vi "MegaAwesome_8_29_12c_JW.vi"() -> ()   [LabVIEW 2011]
uses:
  MegaAwesome_States.ctl
  <vilib>/Utility/file.llb/Read From Spreadsheet File (string).vi
  <vilib>/Utility/file.llb/Write To Spreadsheet File (string).vi
panel:
  in  "Index-Sat":dbl=5.0
  in  "Index-Lin":dbl=5.0
  in  "IndexLog-Lin":dbl=5.0
  in  "IndexLog-Sat":dbl=5.0 caption="Num Pts"
  out "Lin Id-Log Used":dbl[](array[numeric])
  out "Lin-Vg Array-Log Used":dbl[](array[numeric])
  out "Total Width":dbl
  out "Image Preview":T1(plugin-control)
  in  "New: Comments":string
  out "Save Array":string[][](array[string])
  out "Folder Index":i32 caption="Length"
  out "Sat Id-Used":dbl[](array[numeric])
  out "Sat Vg Array-Used":dbl[](array[numeric])
  out "Vg Array-Log-Used":dbl[](array[numeric])
  out "Sat Id-Log-Used":dbl[](array[numeric])
  out "Lin Id-Used":dbl[](array[numeric])
  out "Lin-Vg Array-Used":dbl[](array[numeric])
  out "Lin Vd":dbl
  out "Recorded Prop":T2
  out "Current State":T3
  in  "Main Tab Control":T4(tab)
  in  "Image Folder":path
  out "Image File":path=path "D:/UserData/Desktop/Jeremy/WFU/Research/Programs/VI mods/Image Not Found.png"
  in  "Transfer File":path
  out "Transfer Folder":path
  out "Fabrication Prop":T5
  in  "Manual Controls":T6
  in  "File Controls":T7
  out "Date Recorded":string="Date Recorded" caption="Measured"
  out "Data Name:":string
  out "Image Name":string
  out "Index":string
  out "Date Created":string caption="Fabricated"
  in  "Comments:":string
  out "Rec: Length":dbl caption="Length" format="%#_3g"
  out "Rec: Width":dbl caption="Width" format="%#_4g"
  out "Rec: Dielectric (d)":dbl caption="Dielectric (d)" format="%#_3g"
  in  "New: Dielectric":dbl
  in  "New: Length":dbl
  in  "New: Width":dbl
  out "Rec: Temp":dbl caption="Sample Temp" format="%.1f"
  in  "New: Temp":dbl format="%.1f"
  in  "Independant Variable":string(combo)="Length (um):"
  out "Image Out":T1(plugin-control)
  in  "Num Pts":dbl=5.0
  in  "Num Pts Log":dbl=5.0 caption="Num Pts"
  out "Recorded Values Cluster":T8
  out "Calculated Values Cluster":T8 caption="Recorded Values Cluster"
  out "Re-Calculated Values Cluster":T8 caption="Recorded Values Cluster"
  in  "Origin Project File":path=path "\\\\acad1\\physics/Jurchescu-group/JW-PD/Group Library/Origin Project Files/DeviceData_8_10_12a_JW.opj"
  in  "No Image File":path=path "\\\\acad1\\physics/Jurchescu-group/JW-PD/Mega Awesome/Image Not Found.png"
  in  "Room Temp":dbl=294.0
  # "Image Location"
  # "Recorded"
  # "Calculated"
  # "Re-Calculated"
  # "Manual"
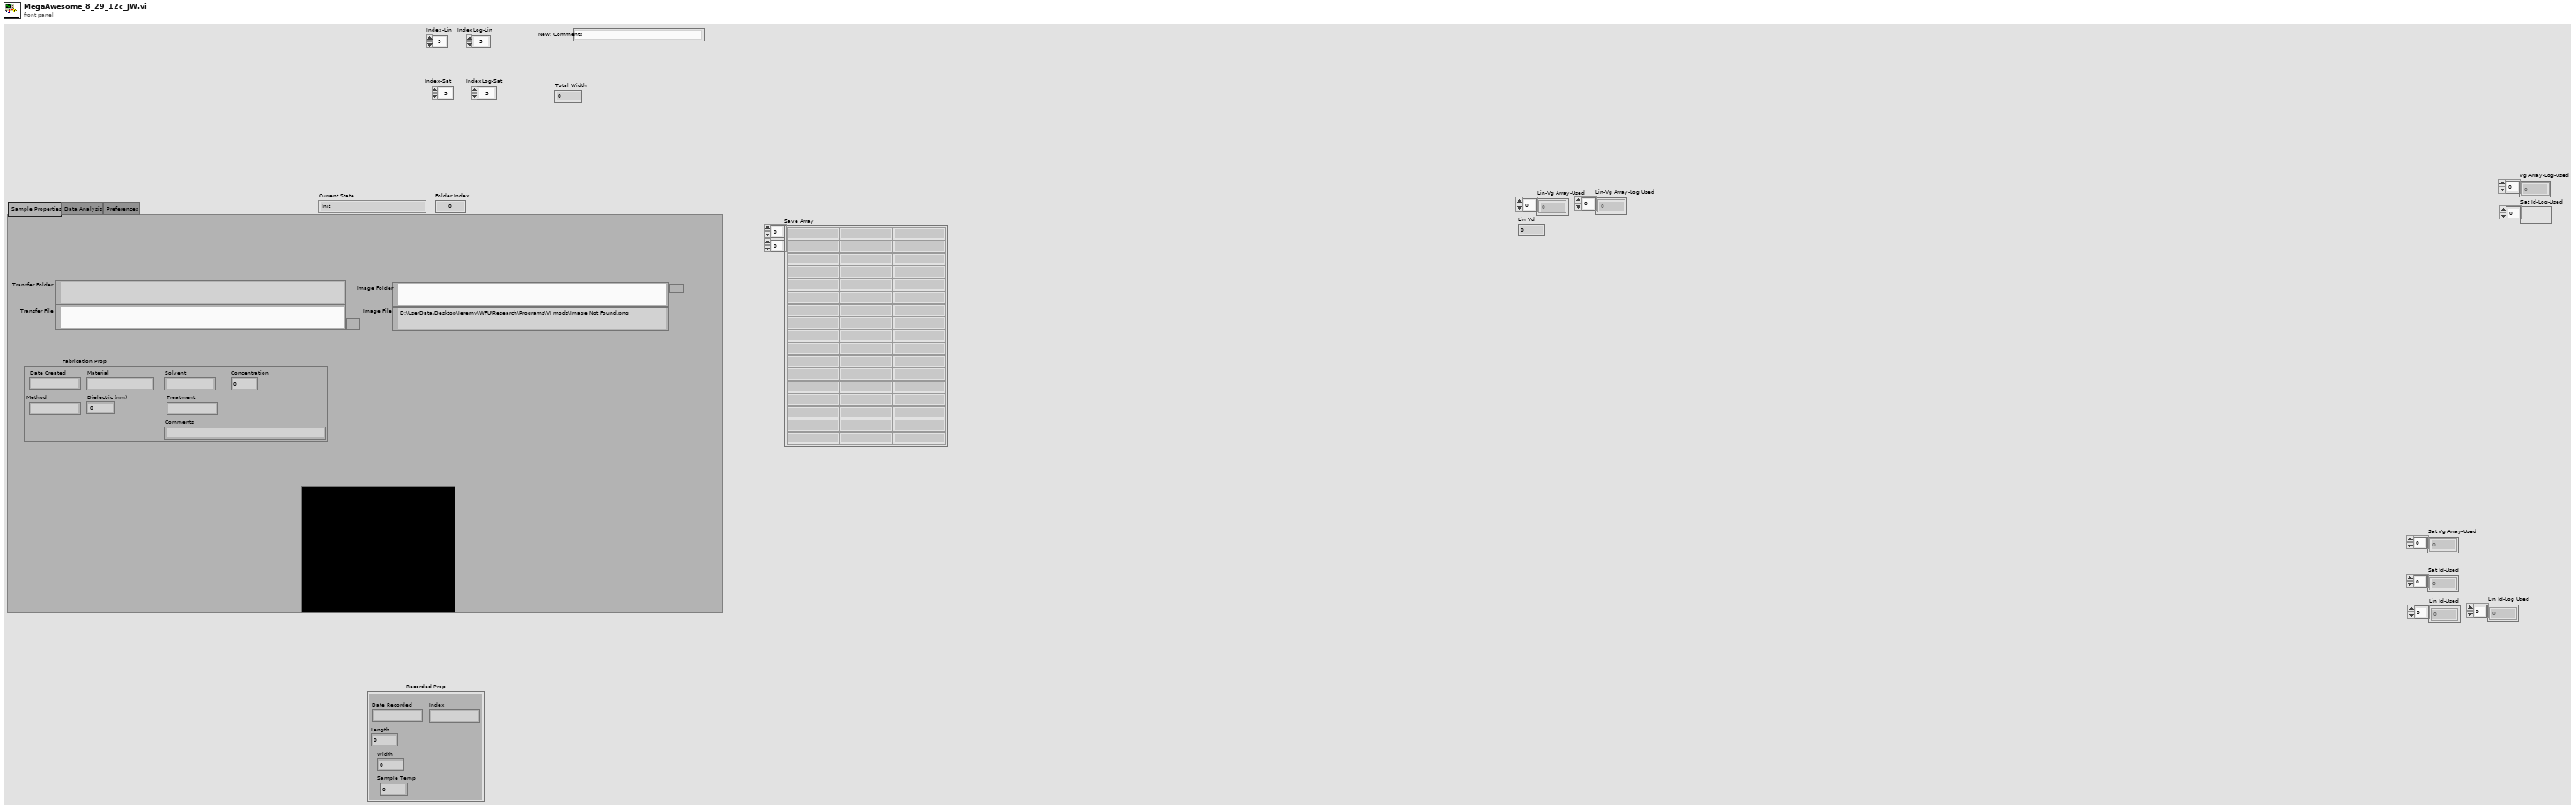
[diagram p1: front panel]
types:
  T1 = typedef "IMAQ Image.ctl" = refnum<image>
  T2 = cluster{"Date Recorded":string, "Index":string, "Length":dbl, "Width":dbl, "Sample Temp":dbl}
  T3 = typedef "MegaAwesome_States.ctl" = enum16{"Init", "File Missing", "No Event", "Read Data", "Calculated Values", "Re-Calculated Values", "Next File", "Previous File", "Discard File", "Save", "Save Lines", "Export", "Exit"}
  T4 = enum32{"Sample Properties", "Data Analysis", "Preferences"}
  T5 = cluster{"Date Created":string, "Material":string, "Solvent":string, "Concentration":dbl, "Method":string, "Dielectric (nm)":dbl, "Treatment":string, "Comments":string}
  T6 = cluster{"Manual-Temp":bool, "Manual-Width":bool, "Manuel-Length":bool, "Manuel-Dielectric":bool, "Manual Comments":bool}
  T7 = cluster{"Previous File":bool, "Discard ":bool, "Save Lines":bool, "Close":bool, "Next File ":bool, "Save":bool, "Save Next":bool, "Export":bool}
  T8 = cluster{"Mobility-Sat":dbl, "Moblitity-Lin":dbl, "On/Off":dbl, "Off Current":dbl, "Vt-Sat":dbl, "STS":dbl, "Trap Density-VT":dbl, "Trap Density-STS":dbl}
  T9 = cluster{"Sat Vg Used":dbl[], "Sat Sqrt(Id) Used ":dbl[], "Lin Vg Used":dbl[], "Lin Sqrt(Id) Used":dbl[], "Index-Lin":dbl, "Index-Sat":dbl}
  T10 = cluster{"Mobility-Sat":dbl, "Vt-Sat":dbl, "Mobility-Lin":dbl, "Vt-Lin":dbl, "Off I-Sat":dbl, "On/Off I-Sat":dbl}
  T11 = cluster{"Sat Vg Used":dbl[], "Sat Log(Id) Used":dbl[], "Lin Vg Used":dbl[], "Lin Log(Id) Used":dbl[], "STS Index-Sat":dbl, "STS Index-Lin":dbl}
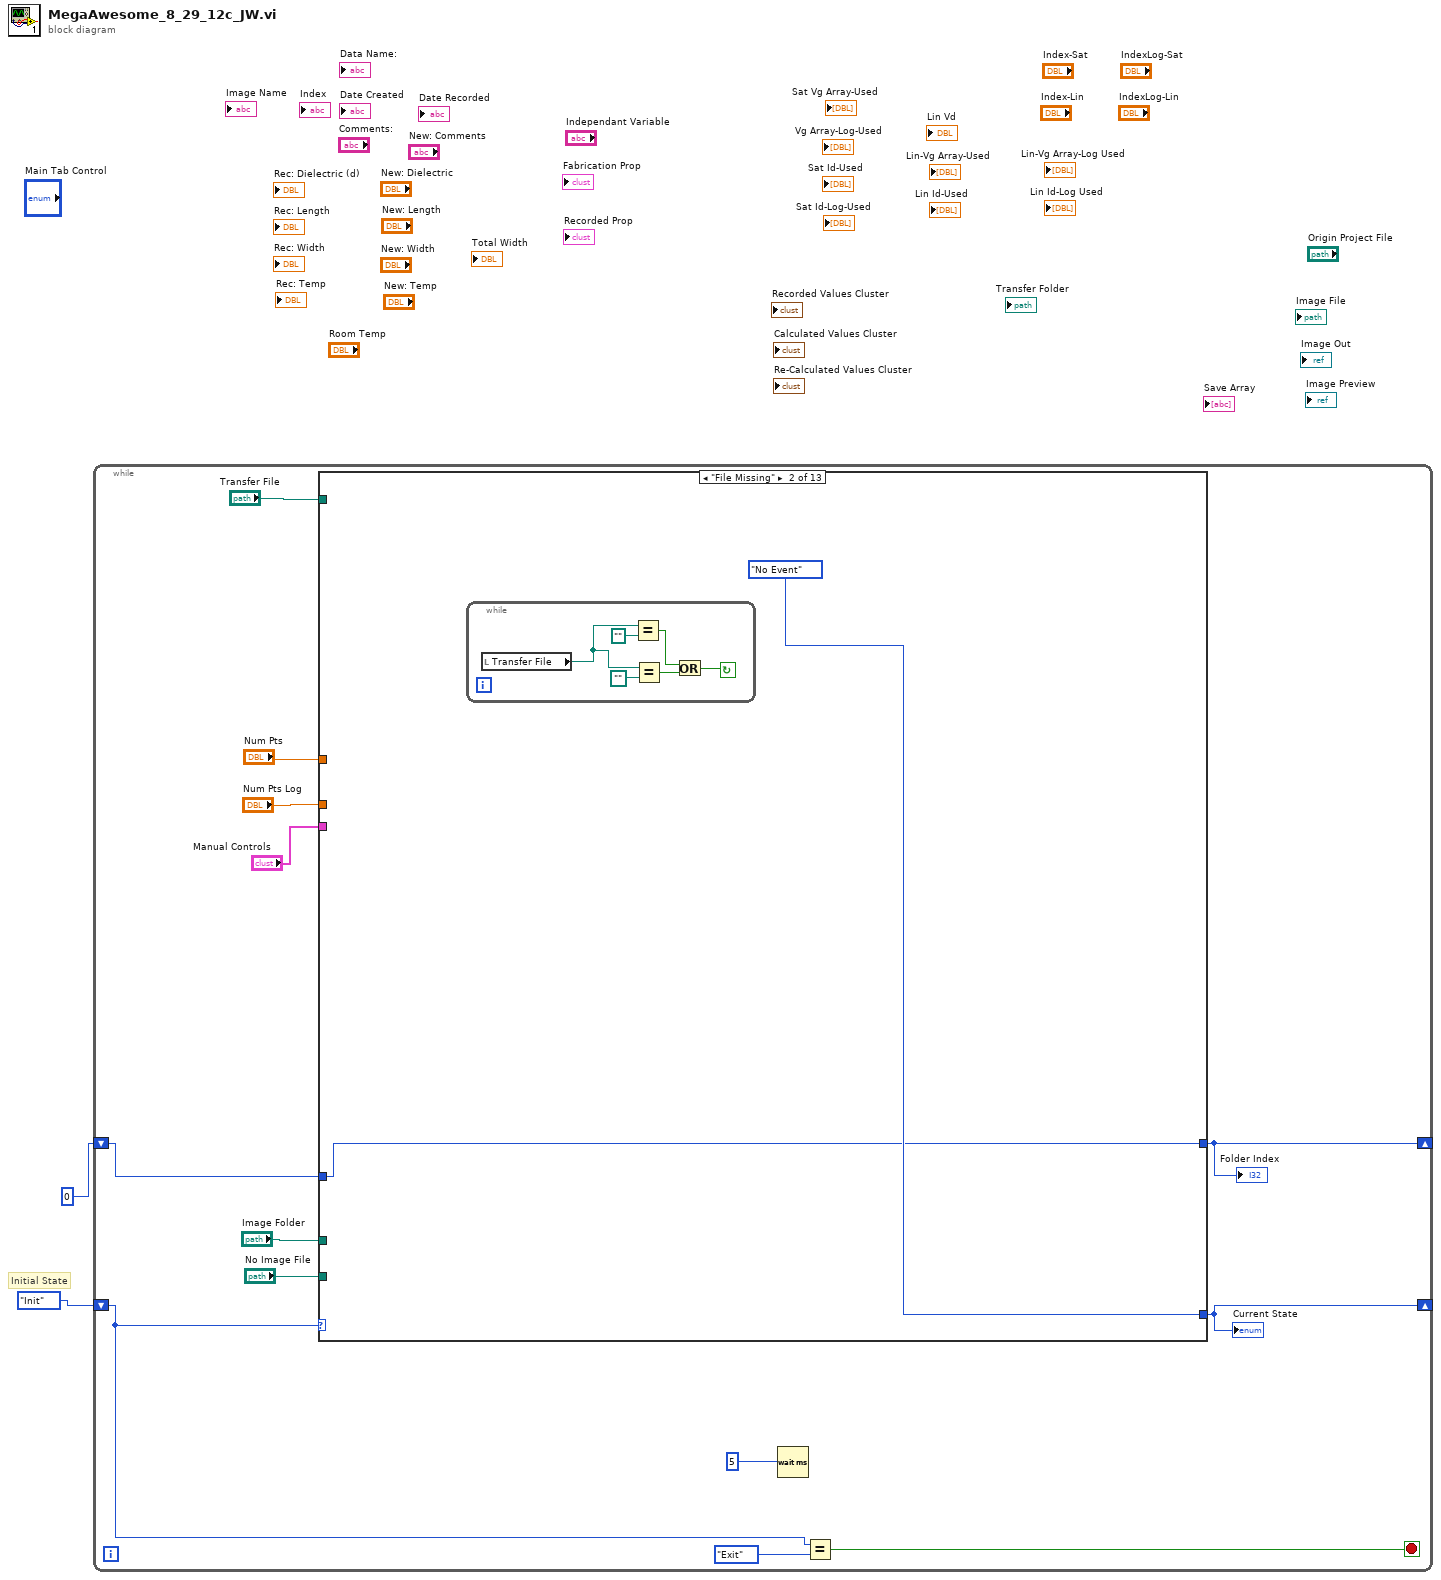
[diagram p0: block diagram]
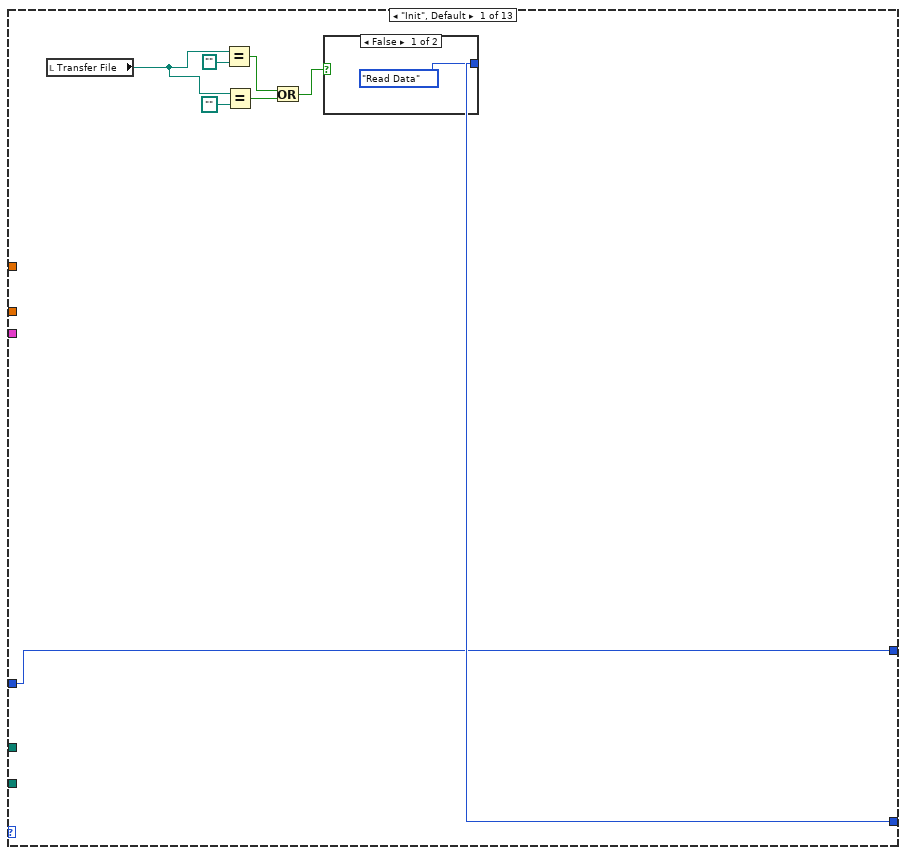
[diagram p2: hidden frame]
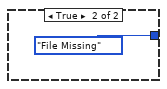
[diagram p3: hidden frame]
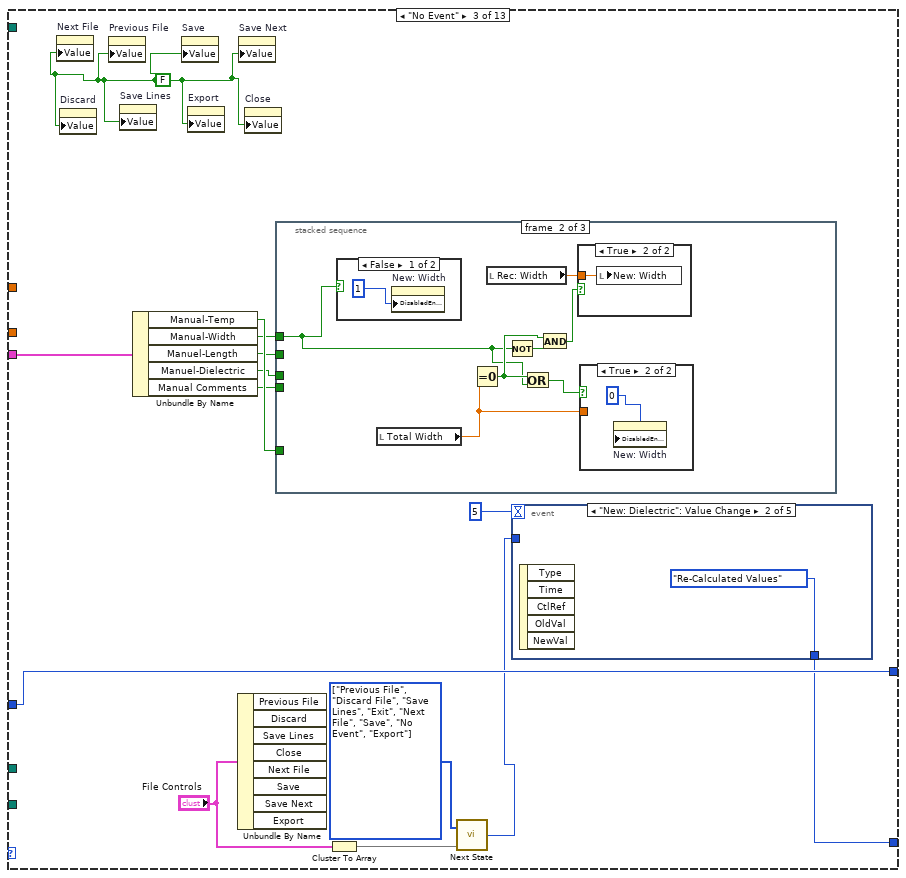
[diagram p4: hidden frame]
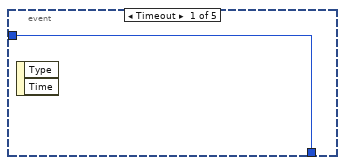
[diagram p5: hidden frame]
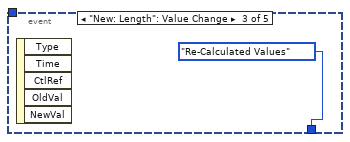
[diagram p6: hidden frame]
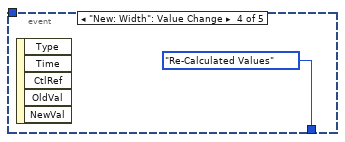
[diagram p7: hidden frame]
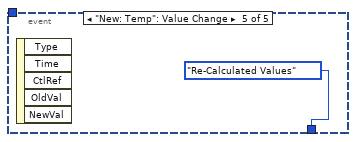
[diagram p8: hidden frame]
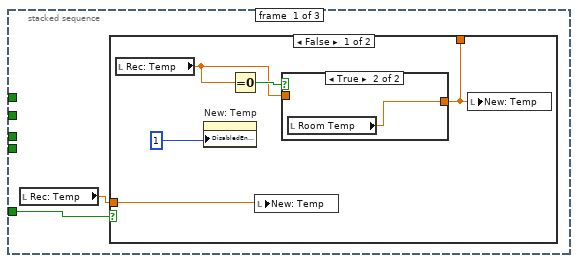
[diagram p9: hidden frame]
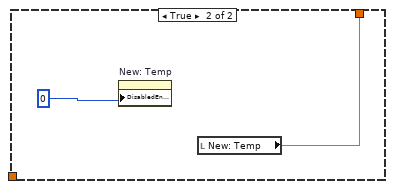
[diagram p11: hidden frame]
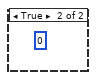
[diagram p12: hidden frame]
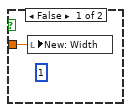
[diagram p14: hidden frame]
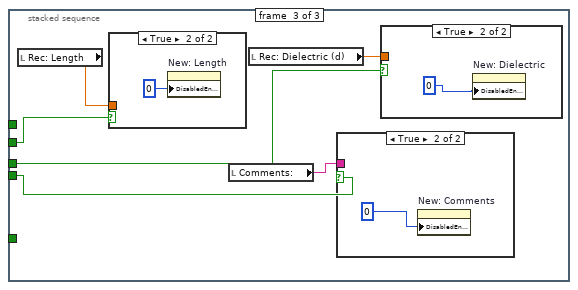
[diagram p15: hidden frame]
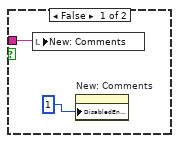
[diagram p16: hidden frame]
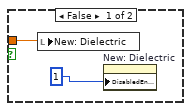
[diagram p17: hidden frame]
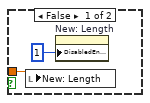
[diagram p18: hidden frame]
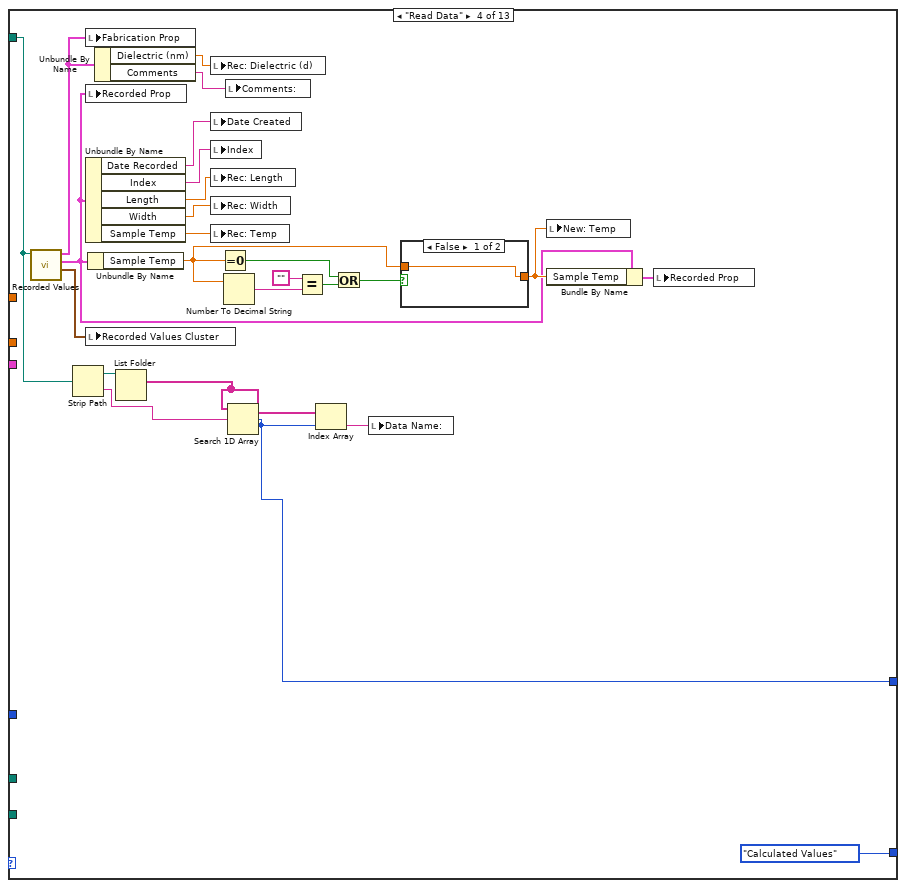
[diagram p19: hidden frame]
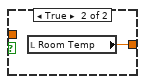
[diagram p20: hidden frame]
diagram:
  # "Initial State"
  n1 = while {
    shift-right: [w12] -> _
    shift-left: MegaAwesome_States."Init" -> [w14]
    shift-right: [w5] -> _
    shift-left: 0 -> [w6]
    stop <- w15 stop-if-true
    n2 = case shown="\"File Missing\"" w14 {
      selector: w14 -> [_ _ _ _ _ _ _ w210 _ _ _ _ _]
      tunnel: [w17 MegaAwesome_States."No Event" w35 MegaAwesome_States."Calculated Values" MegaAwesome_States."Re-Calculated Values" MegaAwesome_States."No Event" MegaAwesome_States."Read Data" w210 MegaAwesome_States."Read Data" MegaAwesome_States."No Event" w235 MegaAwesome_States."No Event" MegaAwesome_States."No Event"] -> w12
      tunnel: "Transfer File" -> [_ _ _ w96 w135 _ w203 _ w217 _ w240 _ _]
      tunnel: "Num Pts" -> [_ _ _ _ w139 _ _ _ _ _ _ _ _]
      tunnel: "Num Pts Log" -> [_ _ _ _ w138 _ _ _ _ _ _ _ _]
      tunnel: "Image Folder" -> [_ _ _ _ w134 _ _ _ _ _ _ _ _]
      tunnel: "No Image File" -> [_ _ _ _ w133 _ _ _ _ _ _ _ _]
      tunnel: [w16 w26 w43 w90 w132 w163 w188 w209 w215 w233 w241 w752 w754] -> w5
      tunnel: w6 -> [w16 w26 w43 _ w132 w163 w189 w209 w216 w233 w241 w752 w754]
      tunnel: "Manual Controls" -> [_ _ w37 _ _ _ _ _ _ _ w239 _ _]
      frame "Init", Default {
        n3 = local read "Transfer File"() -> (w18:path)
        n4 = Equal?(x=w18, y=path "") -> (x = y?=w21:bool)
        n5 = Equal?(x=w18, y=path "") -> (x = y?=w20:bool)
        n6 = Or(x=w21, y=w20) -> (x .or. y?=w23:bool)
        n7 = case shown="False" w23 {
          tunnel: [MegaAwesome_States."Read Data" MegaAwesome_States."File Missing"] -> w17
          frame False {
          }
          frame True {
          }
        }
      }
      frame "File Missing" {
        n8 = while {
          stop <- w28 continue-if-true
          n9 = local read "Transfer File"() -> (w29:path)
          n10 = Equal?(x=w29, y=path "") -> (x = y?=w31:bool)
          n11 = Equal?(x=w29, y=path "") -> (x = y?=w32:bool)
          n12 = Or(x=w31, y=w32) -> (x .or. y?=w28:bool)
        }
      }
      frame "No Event" {
        w46 = T3[] [enum."Previous File", enum."Discard File", enum."Save Lines", enum."Exit", enum."Next File", enum."Save", enum."No Event", enum."Export"] items=["Init", "File Missing", "No Event", "Read Data", "Calculated Values", "Re-Calculated Values", "Next File", "Previous File", "Discard File", "Save", "Save Lines", "Export", "Exit"]
        w47 = FALSE
        n13 = property on="Next File" class="Bool (strict)"("Value"=w47) -> ()  [unwired: 2 in, 2 out]
        n14 = property on="Discard" class="Bool (strict)"("Value"=w47) -> ()  [unwired: 2 in, 2 out]
        n15 = property on="Previous File" class="Bool (strict)"("Value"=w47) -> ()  [unwired: 2 in, 2 out]
        n16 = property on="Save Lines" class="Bool (strict)"("Value"=w47) -> ()  [unwired: 2 in, 2 out]
        n17 = Unbundle By Name(w37) -> ("Manual-Temp"=w42:bool, "Manual-Width"=w41:bool, "Manuel-Length"=w40:bool, "Manuel-Dielectric"=w39:bool, "Manual Comments"=w38:bool)
        n18 = property on="Save" class="Bool (strict)"("Value"=w47) -> ()  [unwired: 2 in, 2 out]
        n19 = property on="Export" class="Bool (strict)"("Value"=w47) -> ()  [unwired: 2 in, 2 out]
        n20 = Unbundle By Name("File Controls") -> ()  [unwired: 8 out]
        n21 = property on="Save Next" class="Bool (strict)"("Value"=w47) -> ()  [unwired: 2 in, 2 out]
        n22 = property on="Close" class="Bool (strict)"("Value"=w47) -> ()  [unwired: 2 in, 2 out]
        n23 = stacked-sequence {
          tunnel: w42 -> [w54 _ _]
          tunnel: w41 -> [_ w64 _]
          tunnel: w40 -> [_ _ w79]
          tunnel: w39 -> [_ _ w76]
          tunnel: w38 -> [_ _ w75]
          frame #0 {
            n24 = local read "Rec: Temp"() -> (w53:dbl)
            n25 = case shown="False" w54 {
              tunnel: w53 -> [w59 _]
              tunnel: [w56 w63] -> _
              frame False {
                n26 = local read "Rec: Temp"() -> (w57:dbl)
                n27 = property on="New: Temp" class="DigNum (strict)"("DisabledEnum"=1) -> ()  [unwired: 2 in, 2 out]
                n28 = Equal To 0?(x=w57) -> (x = 0?=w58:bool)
                n29 = local write "New: Temp"(w59) -> ()
                n30 = case shown="True" w58 {
                  tunnel: [w60 w61] -> w56
                  tunnel: w57 -> [w60 _]
                  frame False {
                  }
                  frame True {
                    n31 = local read "Room Temp"() -> (w61:dbl)
                  }
                }
                n32 = local write "New: Temp"(w56) -> ()
              }
              frame True {
                n33 = property on="New: Temp" class="DigNum (strict)"("DisabledEnum"=0) -> ()  [unwired: 2 in, 2 out]
                n34 = local read "New: Temp"() -> (w63:dbl)
              }
            }
          }
          frame #1 {
            n35 = case shown="False" w64 {
              frame False {
                n36 = property on="New: Width" class="DigNum (strict)"("DisabledEnum"=1) -> ()  [unwired: 2 in, 2 out]
              }
              frame True {
                (unwired) 0
              }
            }
            n37 = local read "Total Width"() -> (w70:dbl)
            n38 = Equal To 0?(x=w70) -> (x = 0?=w67:bool)
            n39 = local read "Rec: Width"() -> (w68:dbl)
            n40 = Not(x=w64) -> (.not. x?=w66:bool)
            n41 = Or(x=w67, y=w64) -> (x .or. y?=w69:bool)
            n42 = And(x=w67, y=w66) -> (x .and. y?=w65:bool)
            n43 = case shown="True" w65 {
              tunnel: w68 -> [_ w72]
              frame False {
              }
              frame True {
                n44 = local write "New: Width"(w72) -> ()
              }
            }
            n45 = case shown="True" w69 {
              tunnel: w70 -> [w73 _]
              frame False {
                (unwired) 1
                n46 = local write "New: Width"(w73) -> ()
              }
              frame True {
                n47 = property on="New: Width" class="DigNum (strict)"("DisabledEnum"=0) -> ()  [unwired: 2 in, 2 out]
              }
            }
          }
          frame #2 {
            n48 = local read "Rec: Length"() -> (w80:dbl)
            n49 = case shown="True" w79 {
              tunnel: w80 -> [w88 _]
              frame False {
                n50 = local write "New: Length"(w88) -> ()
                n51 = property on="New: Length" class="DigNum (strict)"("DisabledEnum"=1) -> ()  [unwired: 2 in, 2 out]
              }
              frame True {
                n52 = property on="New: Length" class="DigNum (strict)"("DisabledEnum"=0) -> ()  [unwired: 2 in, 2 out]
              }
            }
            n53 = local read "Comments:"() -> (w77:string)
            n54 = local read "Rec: Dielectric (d)"() -> (w78:dbl)
            n55 = case shown="True" w75 {
              tunnel: w77 -> [w82 _]
              frame False {
                n56 = local write "New: Comments"(w82) -> ()
                n57 = property on="New: Comments" class="Str"("DisabledEnum"=1) -> ()  [unwired: 2 in, 2 out]
              }
              frame True {
                n58 = property on="New: Comments" class="Str"("DisabledEnum"=0) -> ()  [unwired: 2 in, 2 out]
              }
            }
            n59 = case shown="True" w76 {
              tunnel: w78 -> [w85 _]
              frame False {
                n60 = local write "New: Dielectric"(w85) -> ()
                n61 = property on="New: Dielectric" class="DigNum (strict)"("DisabledEnum"=1) -> ()  [unwired: 2 in, 2 out]
              }
              frame True {
                n62 = property on="New: Dielectric" class="DigNum (strict)"("DisabledEnum"=0) -> ()  [unwired: 2 in, 2 out]
              }
            }
          }
        }
        n63 = Cluster To Array(cluster="File Controls") -> (array=w44:bool[])
        n64 = call "Next State.vi"("Buttons []"=w44, "States []"=w46) -> ("Enum"=w36:T3)
        n65 = event shown="[1] \"New: Dielectric\": Value Change" {
          selector: _ -> [_ _ _ _ _]
          dyn-events: _ -> [_ _ _ _ _]
          timeout: 5 -> [_ _ _ _ _]
          tunnel: w36 -> [w48 _ _ _ _]
          tunnel: [w48 MegaAwesome_States."Re-Calculated Values" MegaAwesome_States."Re-Calculated Values" MegaAwesome_States."Re-Calculated Values" MegaAwesome_States."Re-Calculated Values"] -> w35
          event Timeout {
            n66 = event-data() -> ()  [unwired: 1 in, 2 out]
          }
          event "New: Dielectric": Value Change {
            n67 = event-data() -> ()  [unwired: 1 in, 5 out]
          }
          event "New: Length": Value Change {
            n68 = event-data() -> ()  [unwired: 1 in, 5 out]
          }
          event "New: Width": Value Change {
            n69 = event-data() -> ()  [unwired: 1 in, 5 out]
          }
          event "New: Temp": Value Change {
            n70 = event-data() -> ()  [unwired: 1 in, 5 out]
          }
        }
      }
      frame "Read Data" {
        n71 = call "Recorded Values.vi"("Path"=w96) -> ("Recorded Char"=w114:T8, "Recorded Prop"=w104:T2, "Fabrication Prop"=w98:T5)  [unwired: 8 in]
        n72 = Strip Path(path=w96) -> (stripped path=w97:path, name=w95:string)
        n73 = local write "Fabrication Prop"(w98) -> ()
        n74 = local write "Recorded Prop"(w104) -> ()
        n75 = Unbundle By Name(w104) -> ("Date Recorded"=w103:string, "Index"=w101:string, "Length"=w102:dbl, "Width"=w100:dbl, "Sample Temp"=w99:dbl)
        n76 = local write "Recorded Values Cluster"(w114) -> ()
        n77 = Unbundle By Name(w104) -> ("Sample Temp"=w107:dbl)
        n78 = Unbundle By Name(w98) -> ("Dielectric (nm)"=w92:dbl, "Comments"=w91:string)
        n79 = List Folder(path=w97) -> (filenames=w93:string[])  [unwired: 3 in, 3 out]
        n80 = local write "Rec: Dielectric (d)"(w92) -> ()
        n81 = local write "Date Created"(w103) -> ()
        n82 = local write "Index"(w101) -> ()
        n83 = local write "Rec: Length"(w102) -> ()
        n84 = local write "Rec: Width"(w100) -> ()
        n85 = local write "Rec: Temp"(w99) -> ()
        n86 = Equal To 0?(x=w107) -> (x = 0?=w110:bool)
        n87 = Number To Decimal String(number=w107) -> (decimal integer string=w111:string)  [unwired: 1 in]
        n88 = local write "Comments:"(w91) -> ()
        n89 = Search 1D Array(1D array=w93, element=w95) -> (index of element=w90:i32)  [unwired: 1 in]
        n90 = Equal?(x="", y=w111) -> (x = y?=w109:bool)
        n91 = Index Array(array=w93, index=w90) -> (element=w94:string)
        n92 = Or(x=w110, y=w109) -> (x .or. y?=w108:bool)
        n93 = local write "Data Name:"(w94) -> ()
        n94 = case shown="False" w108 {
          tunnel: [w115 w116] -> w105
          tunnel: w107 -> [w115 _]
          frame False {
          }
          frame True {
            n95 = local read "Room Temp"() -> (w116:dbl)
          }
        }
        n96 = local write "New: Temp"(w105) -> ()
        n97 = Bundle By Name(cluster=w104, "Sample Temp"=w105) -> (w106:T2)
        n98 = local write "Recorded Prop"(w106) -> ()
      }
      frame "Calculated Values" {
        n99 = local read "Fabrication Prop"() -> (w144:T5)
        n100 = local read "Recorded Prop"() -> (w137:T2)
        n101 = disable-structure shown="Disabled" {
          disable-tunnel: w135 -> [w161 _]
          disable-tunnel: w134 -> [w160 _]
          disable-tunnel: w133 -> [w159 _]
          frame Disabled {
            n102 = call "Image from TRF Display.vi"("No Image File"=w159, "Image Folder"=w160, "Transfer File"=w161) -> ("Image Out 2"=w155:T1, "Image Out"=w156:T1, "Image File"=w157:path, "Image Name"=w158:string)  [unwired: 5 in]
            n103 = local write "Image Name"(w158) -> ()
            n104 = local write "Image File"(w157) -> ()
            n105 = local write "Image Out"(w156) -> ()
            n106 = local write "Image Preview"(w155) -> ()
          }
          frame Enabled {
          }
        }
        n107 = local read "Calculated Values Cluster"() -> (w154:T8)
        n108 = call "Mobility-Vt Calculator-File.vi"("NumPts"=w139, "Path"=w135) -> ("Used Points"=w131:T9, "Lin Vd"=w127:dbl, "Output"=w152:T10)  [unwired: 6 in, 1 out]
        n109 = call "STS Calculator-File.vi"("NumPts"=w138, "Path"=w135) -> ("Used Points"=w123:T11, "Ouput"=w147:cluster{"STS-Sat":dbl, "STS-Lin":dbl})  [unwired: 6 in, 2 out]
        n110 = Unbundle By Name(w144) -> ("Dielectric (nm)"=w142:dbl)
        n111 = Unbundle By Name(w137) -> ("Sample Temp"=w136:dbl)
        n112 = Unbundle By Name(w152) -> ("Mobility-Sat"=w151:dbl, "Vt-Sat"=w143:dbl, "Mobility-Lin"=w150:dbl, "Off I-Sat"=w149:dbl, "On/Off I-Sat"=w148:dbl)  [unwired: 1 out]
        n113 = local write "Lin Vd"(w127) -> ()
        n114 = Unbundle By Name(w147) -> ("STS-Sat"=w141:dbl)  [unwired: 1 out]
        n115 = call "Trap Density_VT.vi"("VT"=w143, "Dielectric"=w142) -> ("Trap Density-VT"=w146:dbl)
        n116 = call "Trap Density_STS.vi"("Temp (T) [K]"=w136, "S.T.S. (S)"=w141, "Dielectric"=w142) -> ("Trap Density (N)"=w145:dbl)  [unwired: 8 in]
        n117 = Bundle By Name(cluster=w154, "Mobility-Sat"=w151, "Moblitity-Lin"=w150, "On/Off"=w148, "Off Current"=w149, "Vt-Sat"=w143, "STS"=w141, "Trap Density-VT"=w146, "Trap Density-STS"=w145) -> (w153:T8)
        n118 = Unbundle By Name(w131) -> ("Sat Vg Used"=w130:dbl[], "Sat Sqrt(Id) Used"=w129:dbl[], "Lin Vg Used"=w128:dbl[], "Lin Sqrt(Id) Used"=w126:dbl[], "Index-Lin"=w124:dbl, "Index-Sat"=w125:dbl)
        n119 = Unbundle By Name(w123) -> ("Sat Vg Used"=w120:dbl[], "Sat Log(Id) Used"=w119:dbl[], "Lin Vg Used"=w118:dbl[], "Lin Log(Id) Used"=w117:dbl[], "STS Index-Sat"=w122:dbl, "STS Index-Lin"=w121:dbl)
        n120 = local write "Index-Sat"(w125) -> ()
        n121 = local write "Calculated Values Cluster"(w153) -> ()
        n122 = local write "Sat Vg Array-Used"(w130) -> ()
        n123 = local write "Sat Id-Used"(w129) -> ()
        n124 = local write "Sat Id-Log-Used"(w119) -> ()
        n125 = local write "Lin-Vg Array-Used"(w128) -> ()
        n126 = local write "Index-Lin"(w124) -> ()
        n127 = local write "Lin Id-Used"(w126) -> ()
        n128 = local write "Vg Array-Log-Used"(w120) -> ()
        n129 = local write "IndexLog-Sat"(w122) -> ()
        n130 = local write "Index-Lin"(w121) -> ()
        n131 = local write "Lin-Vg Array-Log Used"(w118) -> ()
        n132 = local write "Lin Id-Log Used"(w117) -> ()
      }
      frame "Re-Calculated Values" {
        n133 = local read "Vg Array-Log-Used"() -> (w170:dbl[])
        n134 = local read "Sat Vg Array-Used"() -> (w178:dbl[])
        n135 = local read "Lin-Vg Array-Used"() -> (w184:dbl[])
        n136 = local read "Sat Id-Log-Used"() -> (w169:dbl[])
        n137 = local read "New: Dielectric"() -> (w182:dbl)
        n138 = local read "New: Dielectric"() -> (w167:dbl)
        n139 = local read "New: Length"() -> (w181:dbl)
        n140 = local read "New: Length"() -> (w177:dbl)
        n141 = local read "New: Width"() -> (w180:dbl)
        n142 = local read "New: Width"() -> (w176:dbl)
        n143 = local read "Lin Id-Used"() -> (w183:dbl[])
        n144 = local read "Sat Id-Used"() -> (w175:dbl[])
        n145 = local read "Re-Calculated Values Cluster"() -> (w186:T8)
        n146 = local read "New: Dielectric"() -> (w166:dbl)
        n147 = local read "New: Temp"() -> (w165:dbl)
        n148 = local read "Lin Vd"() -> (w162:dbl)
        n149 = call "Mobility-Vt-Used Pts_Saturation.vi"("Width"=w176, "Length"=w177, "Dielectric (d)"=w167, "Sat Id Used"=w175, "Vg Used"=w178) -> ("Vt"=w173:dbl, "Mobility"=w174:dbl)  [unwired: 4 in, 1 out]
        n150 = call "STS-Used.vi"("Id Used"=w169, "Vg-Used"=w170) -> ("STS"=w168:dbl)  [unwired: 9 in]
        n151 = call "Mobility-Vt-Used Pts_Linear.vi"("Width"=w180, "Length"=w181, "Vd"=w162, "Dielectric (d)"=w182, "Id Used"=w183, "Vg Used"=w184) -> ("Mobility"=w179:dbl)  [unwired: 3 in, 2 out]
        n152 = call "Trap Density_VT.vi"("VT"=w173, "Dielectric"=w167) -> ("Trap Density-VT"=w172:dbl)
        n153 = call "Trap Density_STS.vi"("Temp (T) [K]"=w165, "S.T.S. (S)"=w168, "Dielectric"=w166) -> ("Trap Density (N)"=w164:dbl)  [unwired: 8 in]
        n154 = Bundle By Name(cluster=w186, "Mobility-Sat"=w174, "Moblitity-Lin"=w179, "Vt-Sat"=w173, "STS"=w168, "Trap Density-VT"=w172, "Trap Density-STS"=w164) -> (w185:T8)
        n155 = local write "Re-Calculated Values Cluster"(w185) -> ()
      }
      frame "Next File" {
        n156 = Strip Path(path=w203) -> (stripped path=w193:path, name=w201:string)
        n157 = local write "Transfer Folder"(w193) -> ()
        n158 = List Folder(path=w193) -> (filenames=w187:string[], error out=w196:errorcluster)  [unwired: 3 in, 2 out]
        n159 = Array Size(array=w187) -> (size(s)=w200:i32)
        n160 = Search 1D Array(1D array=w187, element=w201) -> (index of element=w198:i32)  [unwired: 1 in]
        n161 = Decrement(x=w200) -> (x-1=w199:i32)
        n162 = Equal?(x=w199, y=w198) -> (x = y?=w197:bool)
        n163 = case shown="False" w197 {
          tunnel: w189 -> [w206 _]
          tunnel: [w205 0] -> w188
          tunnel: w196 -> [w204 w207]
          tunnel: [w204 w207] -> _
          frame False {
            n164 = Increment(x=w206) -> (x+1=w205:i32)
          }
          frame True {
          }
        }
        n165 = Path To String(path=w193) -> (string=w194:string)
        n166 = Index Array(array=w187, index=w188) -> (element=w195:string)
        n167 = Concatenate Strings(w194, "\\", w195) -> (w191:string)
        n168 = String To Path(string=w191) -> (path=w190:path)
        n169 = local write "Transfer File"(w190) -> ()
      }
      frame "Exit" {
      }
      frame "Previous File" {
        n170 = Strip Path(path=w217) -> (stripped path=w214:path, name=w226:string)
        n171 = local write "Transfer Folder"(w214) -> ()
        n172 = List Folder(path=w214) -> (filenames=w218:string[], error out=w223:errorcluster)  [unwired: 3 in, 2 out]
        n173 = Array Size(array=w218) -> (size(s)=w212:i32)
        n174 = Search 1D Array(1D array=w218, element=w226) -> (index of element=w225:i32)  [unwired: 1 in]
        n175 = Decrement(x=w212) -> (x-1=w211:i32)
        n176 = Equal To 0?(x=w225) -> (x = 0?=w224:bool)
        n177 = case shown="False" w224 {
          tunnel: w216 -> [w230 _]
          tunnel: [w229 w231] -> w215
          tunnel: w223 -> [w228 w232]
          tunnel: [w228 w232] -> _
          tunnel: w211 -> [_ w231]
          frame False {
            n178 = Decrement(x=w230) -> (x-1=w229:i32)
          }
          frame True {
          }
        }
        n179 = Path To String(path=w214) -> (string=w213:string)
        n180 = Index Array(array=w218, index=w215) -> (element=w222:string)
        n181 = Concatenate Strings(w213, "\\", w222) -> (w220:string)
        n182 = String To Path(string=w220) -> (path=w219:path)
        n183 = local write "Transfer File"(w219) -> ()
      }
      frame "Discard File" {
      }
      frame "Save" {
        n184 = stacked-sequence {
          seq-local: [w245 _] -> [_ w742]
          seq-local: [w244 _] -> [_ w740]
          tunnel: w240 -> [w246 w743]
          frame #0 {
            # "Saves each Re-calculated parameter in sequence"
            n185 = stacked-sequence {
              tunnel: [_ _ _ _ _ _ _ _ _ _ _ _ _ w710] -> w244
              tunnel: w246 -> [w266 _ _ _ _ _ _ _ _ _ _ _ _ _]
              frame #0 {
                n186 = call-poly <vilib>:"Read From Spreadsheet File.vi"("file path (dialog if empty)"=w266) -> ("all rows"=w265:string[][])  [unwired: 6 in, 4 out]
                n187 = Array Size(array=w265) -> (size(s)=w270:i32[])
                n188 = Array Subset(array=w265, index (row)=0, index (col)=0, length (col)=3) -> (w274:string[][])  [unwired: 1 in]
                n189 = Index Array(array=w270, index=0) -> (element=w268:i32)
                n190 = Reshape Array(w274, w268) -> (w267:string[])
                n191 = Search 1D Array(1D array=w267, element="Dielectric (nm):") -> (index of element=w277:i32)  [unwired: 1 in]
                n192 = Equal?(x=w277, y=-1) -> (x = y?=w276:bool)
                n193 = case shown="False" w276 {
                  tunnel: w265 -> [w285 w289]
                  tunnel: w277 -> [w281 _]
                  tunnel: [w280 w289] -> w275
                  frame False {
                    n194 = local read "Rec: Dielectric (d)"() -> (w287:dbl)
                    n195 = Number To Fractional String(number=w287) -> (F-format string=w282:string)  [unwired: 3 in]
                    n196 = Divide(x=w281, y=3) -> (x/y=w284:dbl)
                    n197 = To Word Integer(number=w284) -> (16bit integer=w283:i16)
                    n198 = Replace Array Subset(array=w285, new element=w282, index (row)=w283, index (col)=1) -> (w280:string[][])
                  }
                  frame True {
                  }
                }
                n199 = local write "Save Array"(w275) -> ()
              }
              frame #1 {
                n200 = local read "Save Array"() -> (w291:string[][])
                n201 = Array Size(array=w291) -> (size(s)=w294:i32[])
                n202 = Array Subset(array=w291, index (row)=0, index (col)=0, length (col)=3) -> (w298:string[][])  [unwired: 1 in]
                n203 = Index Array(array=w294, index=0) -> (element=w292:i32)
                n204 = Reshape Array(w298, w292) -> (w290:string[])
                n205 = Search 1D Array(1D array=w290, element="Comments:") -> (index of element=w301:i32)  [unwired: 1 in]
                n206 = Equal?(x=w301, y=-1) -> (x = y?=w300:bool)
                n207 = case shown="False" w300 {
                  tunnel: w291 -> [w309 w312]
                  tunnel: w301 -> [w306 _]
                  tunnel: [w305 w312] -> w299
                  frame False {
                    n208 = local read "New: Comments"() -> (w304:string)
                    n209 = Divide(x=w306, y=3) -> (x/y=w308:dbl)
                    n210 = To Word Integer(number=w308) -> (16bit integer=w307:i16)
                    n211 = Replace Array Subset(array=w309, new element=w304, index (row)=w307, index (col)=1) -> (w305:string[][])
                  }
                  frame True {
                  }
                }
                n212 = local write "Save Array"(w299) -> ()
              }
              frame #2 {
                n213 = local read "Save Array"() -> (w314:string[][])
                n214 = Array Size(array=w314) -> (size(s)=w317:i32[])
                n215 = Array Subset(array=w314, index (row)=0, index (col)=0, length (col)=3) -> (w321:string[][])  [unwired: 1 in]
                n216 = Index Array(array=w317, index=0) -> (element=w315:i32)
                n217 = Reshape Array(w321, w315) -> (w313:string[])
                n218 = Search 1D Array(1D array=w313, element="Length (um):") -> (index of element=w324:i32)  [unwired: 1 in]
                n219 = Equal?(x=w324, y=-1) -> (x = y?=w323:bool)
                n220 = case shown="False" w323 {
                  tunnel: w314 -> [w334 w337]
                  tunnel: w324 -> [w331 _]
                  tunnel: [w330 w337] -> w322
                  frame False {
                    n221 = local read "New: Length"() -> (w327:dbl)
                    n222 = Divide(x=w331, y=3) -> (x/y=w333:dbl)
                    n223 = Format Value(format string="%#g", value (0)=w327) -> (output string=w328:string)  [unwired: 1 in]
                    n224 = To Word Integer(number=w333) -> (16bit integer=w332:i16)
                    n225 = Replace Array Subset(array=w334, new element=w328, index (row)=w332, index (col)=1) -> (w330:string[][])
                  }
                  frame True {
                  }
                }
                n226 = local write "Save Array"(w322) -> ()
              }
              frame #3 {
                n227 = local read "Save Array"() -> (w339:string[][])
                n228 = Array Size(array=w339) -> (size(s)=w344:i32[])
                n229 = Array Subset(array=w339, index (row)=0, index (col)=0, length (col)=3) -> (w340:string[][])  [unwired: 1 in]
                n230 = Index Array(array=w344, index=0) -> (element=w346:i32)
                n231 = Reshape Array(w340, w346) -> (w338:string[])
                n232 = Search 1D Array(1D array=w338, element="Width (um):") -> (index of element=w349:i32)  [unwired: 1 in]
                n233 = Equal?(x=w349, y=-1) -> (x = y?=w348:bool)
                n234 = case shown="False" w348 {
                  tunnel: w349 -> [w357 _]
                  tunnel: w339 -> [w356 w362]
                  tunnel: [w355 w362] -> w347
                  frame False {
                    n235 = local read "New: Width"() -> (w352:dbl)
                    n236 = Divide(x=w357, y=3) -> (x/y=w359:dbl)
                    n237 = To Word Integer(number=w359) -> (16bit integer=w358:i16)
                    n238 = Format Value(format string="%#g", value (0)=w352) -> (output string=w353:string)  [unwired: 1 in]
                    n239 = Replace Array Subset(array=w356, new element=w353, index (row)=w358, index (col)=1) -> (w355:string[][])
                  }
                  frame True {
                  }
                }
                n240 = local write "Save Array"(w347) -> ()
              }
              frame #4 {
                w372 = "Sample Temp (K):"
                n241 = local read "Save Array"() -> (w364:string[][])
                n242 = Array Size(array=w364) -> (size(s)=w369:i32[])
                n243 = Array Subset(array=w364, index (row)=0, index (col)=0, length (col)=3) -> (w365:string[][])  [unwired: 1 in]
                n244 = Index Array(array=w369, index=0) -> (element=w371:i32)
                n245 = Reshape Array(w365, w371) -> (w363:string[])
                n246 = Search 1D Array(1D array=w363, element=w372) -> (index of element=w375:i32)  [unwired: 1 in]
                n247 = Equal?(x=w375, y=-1) -> (x = y?=w374:bool)
                n248 = case shown="False" w374 {
                  tunnel: w364 -> [w384 w398]
                  tunnel: w375 -> [w381 _]
                  tunnel: [w380 w397] -> w373
                  tunnel: w363 -> [_ w400]
                  tunnel: w372 -> [_ w387]
                  frame False {
                    n249 = local read "New: Temp"() -> (w378:dbl)
                    n250 = Divide(x=w381, y=3) -> (x/y=w383:dbl)
                    n251 = Format Value(format string="%#g", value (0)=w378) -> (output string=w377:string)  [unwired: 1 in]
                    n252 = To Word Integer(number=w383) -> (16bit integer=w382:i16)
                    n253 = Replace Array Subset(array=w384, new element=w377, index (row)=w382, index (col)=1) -> (w380:string[][])
                  }
                  frame True {
                    n254 = local read "New: Temp"() -> (w389:dbl)
                    n255 = Search 1D Array(1D array=w400, element="Width (um):") -> (index of element=w394:i32)  [unwired: 1 in]
                    n256 = Divide(x=w394, y=3) -> (x/y=w395:dbl)
                    n257 = To Word Integer(number=w395) -> (16bit integer=w393:i16)
                    n258 = Format Value(format string="%#g", value (0)=w389) -> (output string=w388:string)  [unwired: 1 in]
                    n259 = Build Array(w387, w388) -> (w391:string[])
                    n260 = Increment(x=w393) -> (x+1=w392:i16)
                    n261 = Insert Into Array(array=w398, index (row)=w392, new element=w391) -> (w397:string[][])  [unwired: 1 in]
                  }
                }
                n262 = local write "Save Array"(w373) -> ()
              }
              frame #5 {
                w410 = "Mobility-Sat (cm^2/Vs):"
                n263 = local read "Save Array"() -> (w402:string[][])
                n264 = Array Size(array=w402) -> (size(s)=w407:i32[])
                n265 = Array Subset(array=w402, index (row)=0, index (col)=0, length (col)=3) -> (w403:string[][])  [unwired: 1 in]
                n266 = Index Array(array=w407, index=0) -> (element=w409:i32)
                n267 = Reshape Array(w403, w409) -> (w401:string[])
                n268 = Search 1D Array(1D array=w401, element=w410) -> (index of element=w413:i32)  [unwired: 1 in]
                n269 = Equal?(x=w413, y=-1) -> (x = y?=w412:bool)
                n270 = case shown="False" w412 {
                  tunnel: w402 -> [w423 w433]
                  tunnel: w413 -> [w420 _]
                  tunnel: [w419 w432] -> w411
                  tunnel: w401 -> [_ w430]
                  tunnel: w410 -> [_ w428]
                  frame False {
                    n271 = local read "Re-Calculated Values Cluster"() -> (w416:T8)
                    n272 = Unbundle By Name(w416) -> ("Mobility-Sat"=w415:dbl)
                    n273 = Divide(x=w420, y=3) -> (x/y=w422:dbl)
                    n274 = To Word Integer(number=w422) -> (16bit integer=w421:i16)
                    n275 = Format Value(format string="%#g", value (0)=w415) -> (output string=w417:string)  [unwired: 1 in]
                    n276 = Replace Array Subset(array=w423, new element=w417, index (row)=w421, index (col)=1) -> (w419:string[][])
                  }
                  frame True {
                    n277 = local read "Re-Calculated Values Cluster"() -> (w427:T8)
                    n278 = Unbundle By Name(w427) -> ("Mobility-Sat"=w426:dbl)
                    n279 = Search 1D Array(1D array=w430, element="Mobility (cm^2/Vs):") -> (index of element=w436:i32)  [unwired: 1 in]
                    n280 = Divide(x=w436, y=3) -> (x/y=w437:dbl)
                    n281 = To Word Integer(number=w437) -> (16bit integer=w429:i16)
                    n282 = Format Value(format string="%#g", value (0)=w426) -> (output string=w431:string)  [unwired: 1 in]
                    n283 = Build Array(w428, w431) -> (w435:string[])
                    n284 = Replace Array Subset(array=w433, new element=w435, index (row)=w429) -> (w432:string[][])  [unwired: 1 in]
                  }
                }
                n285 = local write "Save Array"(w411) -> ()
              }
              frame #6 {
                w449 = "Mobility-Lin (cm^2/Vs):"
                n286 = local read "Save Array"() -> (w440:string[][])
                n287 = Array Size(array=w440) -> (size(s)=w446:i32[])
                n288 = Array Subset(array=w440, index (row)=0, index (col)=0, length (col)=3) -> (w442:string[][])  [unwired: 1 in]
                n289 = Index Array(array=w446, index=0) -> (element=w448:i32)
                n290 = Reshape Array(w442, w448) -> (w441:string[])
                n291 = Search 1D Array(1D array=w441, element=w449) -> (index of element=w452:i32)  [unwired: 1 in]
                n292 = Equal?(x=w452, y=-1) -> (x = y?=w451:bool)
                n293 = case shown="True" w451 {
                  tunnel: w440 -> [w462 w470]
                  tunnel: w452 -> [w459 _]
                  tunnel: [w458 w469] -> w450
                  tunnel: w441 -> [_ w468]
                  tunnel: w449 -> [_ w467]
                  frame False {
                    n294 = local read "Re-Calculated Values Cluster"() -> (w455:T8)
                    n295 = Unbundle By Name(w455) -> ("Moblitity-Lin"=w454:dbl)
                    n296 = Divide(x=w459, y=3) -> (x/y=w461:dbl)
                    n297 = To Word Integer(number=w461) -> (16bit integer=w460:i16)
                    n298 = Format Value(format string="%#g", value (0)=w454) -> (output string=w456:string)  [unwired: 1 in]
                    n299 = Replace Array Subset(array=w462, new element=w456, index (row)=w460, index (col)=1) -> (w458:string[][])
                  }
                  frame True {
                    n300 = local read "Re-Calculated Values Cluster"() -> (w466:T8)
                    n301 = Unbundle By Name(w466) -> ("Moblitity-Lin"=w465:dbl)
                    n302 = Search 1D Array(1D array=w468, element="Mobility-Sat (cm^2/Vs):") -> (index of element=w475:i32)  [unwired: 1 in]
                    n303 = Divide(x=w475, y=3) -> (x/y=w476:dbl)
                    n304 = To Word Integer(number=w476) -> (16bit integer=w474:i16)
                    n305 = Format Value(format string="%#g", value (0)=w465) -> (output string=w479:string)  [unwired: 1 in]
                    n306 = Build Array(w467, w479) -> (w472:string[])
                    n307 = Increment(x=w474) -> (x+1=w473:i16)
                    n308 = Insert Into Array(array=w470, index (row)=w473, new element=w472) -> (w469:string[][])  [unwired: 1 in]
                  }
                }
                n309 = local write "Save Array"(w450) -> ()
              }
              frame #7 {
                w489 = "On/Off I-Sat:"
                n310 = local read "Save Array"() -> (w480:string[][])
                n311 = Array Size(array=w480) -> (size(s)=w486:i32[])
                n312 = Array Subset(array=w480, index (row)=0, index (col)=0, length (col)=3) -> (w482:string[][])  [unwired: 1 in]
                n313 = Index Array(array=w486, index=0) -> (element=w488:i32)
                n314 = Reshape Array(w482, w488) -> (w481:string[])
                n315 = Search 1D Array(1D array=w481, element=w489) -> (index of element=w492:i32)  [unwired: 1 in]
                n316 = Equal?(x=w492, y=-1) -> (x = y?=w491:bool)
                n317 = case shown="True" w491 {
                  tunnel: w480 -> [w502 w511]
                  tunnel: w492 -> [w499 _]
                  tunnel: [w498 w512] -> w490
                  tunnel: w481 -> [_ w509]
                  tunnel: w489 -> [_ w507]
                  frame False {
                    n318 = local read "Re-Calculated Values Cluster"() -> (w495:T8)
                    n319 = Divide(x=w499, y=3) -> (x/y=w501:dbl)
                    n320 = Unbundle By Name(w495) -> ("On/Off"=w494:dbl)
                    n321 = To Word Integer(number=w501) -> (16bit integer=w500:i16)
                    n322 = Format Value(format string="%#g", value (0)=w494) -> (output string=w496:string)  [unwired: 1 in]
                    n323 = Replace Array Subset(array=w502, new element=w496, index (row)=w500, index (col)=1) -> (w498:string[][])
                  }
                  frame True {
                    n324 = local read "Re-Calculated Values Cluster"() -> (w506:T8)
                    n325 = Unbundle By Name(w506) -> ("On/Off"=w505:dbl)
                    n326 = Search 1D Array(1D array=w509, element="On/Off Current:") -> (index of element=w515:i32)  [unwired: 1 in]
                    n327 = Divide(x=w515, y=3) -> (x/y=w516:dbl)
                    n328 = To Word Integer(number=w516) -> (16bit integer=w508:i16)
                    n329 = Format Value(format string="%#g", value (0)=w505) -> (output string=w510:string)  [unwired: 1 in]
                    n330 = Build Array(w507, w510) -> (w514:string[])
                    n331 = Replace Array Subset(array=w511, new element=w514, index (row)=w508) -> (w512:string[][])  [unwired: 1 in]
                  }
                }
                n332 = local write "Save Array"(w490) -> ()
              }
              frame #8 {
                w528 = "Off I-Sat (A):"
                n333 = local read "Save Array"() -> (w519:string[][])
                n334 = Array Size(array=w519) -> (size(s)=w525:i32[])
                n335 = Array Subset(array=w519, index (row)=0, index (col)=0, length (col)=3) -> (w521:string[][])  [unwired: 1 in]
                n336 = Index Array(array=w525, index=0) -> (element=w527:i32)
                n337 = Reshape Array(w521, w527) -> (w520:string[])
                n338 = Search 1D Array(1D array=w520, element=w528) -> (index of element=w531:i32)  [unwired: 1 in]
                n339 = Equal?(x=w531, y=-1) -> (x = y?=w530:bool)
                n340 = case shown="True" w530 {
                  tunnel: w519 -> [w541 w549]
                  tunnel: w531 -> [w538 _]
                  tunnel: [w537 w548] -> w529
                  tunnel: w520 -> [_ w547]
                  tunnel: w528 -> [_ w546]
                  frame False {
                    n341 = local read "Re-Calculated Values Cluster"() -> (w534:T8)
                    n342 = Unbundle By Name(w534) -> ("Off Current"=w533:dbl)
                    n343 = Divide(x=w538, y=3) -> (x/y=w540:dbl)
                    n344 = Format Value(format string="%#g", value (0)=w533) -> (output string=w535:string)  [unwired: 1 in]
                    n345 = To Word Integer(number=w540) -> (16bit integer=w539:i16)
                    n346 = Replace Array Subset(array=w541, new element=w535, index (row)=w539, index (col)=1) -> (w537:string[][])
                  }
                  frame True {
                    n347 = local read "Re-Calculated Values Cluster"() -> (w545:T8)
                    n348 = Unbundle By Name(w545) -> ("Off Current"=w544:dbl)
                    n349 = Search 1D Array(1D array=w547, element="On/Off I-Sat:") -> (index of element=w554:i32)  [unwired: 1 in]
                    n350 = Divide(x=w554, y=3) -> (x/y=w555:dbl)
                    n351 = To Word Integer(number=w555) -> (16bit integer=w553:i16)
                    n352 = Format Value(format string="%#g", value (0)=w544) -> (output string=w558:string)  [unwired: 1 in]
                    n353 = Build Array(w546, w558) -> (w551:string[])
                    n354 = Increment(x=w553) -> (x+1=w552:i16)
                    n355 = Insert Into Array(array=w549, index (row)=w552, new element=w551) -> (w548:string[][])  [unwired: 1 in]
                  }
                }
                n356 = local write "Save Array"(w529) -> ()
              }
              frame #9 {
                w560 = "Vt-Sat (V):"
                n357 = local read "Save Array"() -> (w561:string[][])
                n358 = Array Size(array=w561) -> (size(s)=w566:i32[])
                n359 = Array Subset(array=w561, index (row)=0, index (col)=0, length (col)=3) -> (w562:string[][])  [unwired: 1 in]
                n360 = Index Array(array=w566, index=0) -> (element=w568:i32)
                n361 = Reshape Array(w562, w568) -> (w559:string[])
                n362 = Search 1D Array(1D array=w559, element=w560) -> (index of element=w571:i32)  [unwired: 1 in]
                n363 = Equal?(x=w571, y=-1) -> (x = y?=w570:bool)
                n364 = case shown="False" w570 {
                  tunnel: w561 -> [w580 w590]
                  tunnel: w571 -> [w576 _]
                  tunnel: [w575 w589] -> w569
                  tunnel: w560 -> [_ w588]
                  tunnel: w559 -> [_ w587]
                  frame False {
                    n365 = local read "Re-Calculated Values Cluster"() -> (w574:T8)
                    n366 = Unbundle By Name(w574) -> ("Vt-Sat"=w573:dbl)
                    n367 = Divide(x=w576, y=3) -> (x/y=w579:dbl)
                    n368 = To Word Integer(number=w579) -> (16bit integer=w578:i16)
                    n369 = Number To Fractional String(number=w573) -> (F-format string=w577:string)  [unwired: 3 in]
                    n370 = Replace Array Subset(array=w580, new element=w577, index (row)=w578, index (col)=1) -> (w575:string[][])
                  }
                  frame True {
                    n371 = local read "Re-Calculated Values Cluster"() -> (w584:T8)
                    n372 = Unbundle By Name(w584) -> ("Vt-Sat"=w583:dbl)
                    n373 = Search 1D Array(1D array=w587, element="Threshold V (V):") -> (index of element=w586:i32)  [unwired: 1 in]
                    n374 = Divide(x=w586, y=3) -> (x/y=w593:dbl)
                    n375 = To Word Integer(number=w593) -> (16bit integer=w585:i16)
                    n376 = Format Value(format string="%#g", value (0)=w583) -> (output string=w596:string)  [unwired: 1 in]
                    n377 = Build Array(w588, w596) -> (w592:string[])
                    n378 = Replace Array Subset(array=w590, new element=w592, index (row)=w585) -> (w589:string[][])  [unwired: 1 in]
                  }
                }
                n379 = local write "Save Array"(w569) -> ()
              }
              frame #10 {
                n380 = disable-structure shown="Disabled" {
                  frame Disabled {
                    n381 = local read "Save Array"() -> (w597:string[][])
                    n382 = Array Size(array=w597) -> (size(s)=w603:i32[])
                    n383 = Array Subset(array=w597, index (row)=0, index (col)=0, length (col)=3) -> (w599:string[][])  [unwired: 1 in]
                    n384 = Index Array(array=w603, index=0) -> (element=w605:i32)
                    n385 = Reshape Array(w599, w605) -> (w598:string[])
                    n386 = Search 1D Array(1D array=w598, element="VT-Lin (V):") -> (index of element=w608:i32)  [unwired: 1 in]
                    n387 = Equal?(x=w608, y=-1) -> (x = y?=w607:bool)
                    n388 = case shown="False" w607 {
                      tunnel: w597 -> [w617 w620]
                      tunnel: w608 -> [w614 _]
                      tunnel: [w613 w620] -> w606
                      frame False {
                        n389 = Divide(x=w614, y=3) -> (x/y=w616:dbl)
                        n390 = To Word Integer(number=w616) -> (16bit integer=w615:i16)
                        n391 = Format Value(format string="%#g") -> (output string=w611:string)  [unwired: 2 in]
                        n392 = Replace Array Subset(array=w617, new element=w611, index (row)=w615, index (col)=1) -> (w613:string[][])
                      }
                      frame True {
                      }
                    }
                    n393 = local write "Save Array"(w606) -> ()
                  }
                  frame Enabled {
                  }
                }
              }
              frame #11 {
                w621 = "STS-Sat (V/decade):"
                n394 = local read "Save Array"() -> (w623:string[][])
                n395 = Array Size(array=w623) -> (size(s)=w628:i32[])
                n396 = Array Subset(array=w623, index (row)=0, index (col)=0, length (col)=3) -> (w624:string[][])  [unwired: 1 in]
                n397 = Index Array(array=w628, index=0) -> (element=w630:i32)
                n398 = Reshape Array(w624, w630) -> (w622:string[])
                n399 = Search 1D Array(1D array=w622, element=w621) -> (index of element=w633:i32)  [unwired: 1 in]
                n400 = Equal?(x=w633, y=-1) -> (x = y?=w632:bool)
                n401 = case shown="True" w632 {
                  tunnel: w623 -> [w643 w651]
                  tunnel: w633 -> [w640 _]
                  tunnel: [w639 w652] -> w631
                  tunnel: w622 -> [_ w650]
                  tunnel: w621 -> [_ w649]
                  frame False {
                    n402 = local read "Re-Calculated Values Cluster"() -> (w635:T8)
                    n403 = Unbundle By Name(w635) -> ("STS"=w636:dbl)
                    n404 = Divide(x=w640, y=3) -> (x/y=w642:dbl)
                    n405 = To Word Integer(number=w642) -> (16bit integer=w641:i16)
                    n406 = Format Value(format string="%#g", value (0)=w636) -> (output string=w637:string)  [unwired: 1 in]
                    n407 = Replace Array Subset(array=w643, new element=w637, index (row)=w641, index (col)=1) -> (w639:string[][])
                  }
                  frame True {
                    n408 = local read "Re-Calculated Values Cluster"() -> (w646:T8)
                    n409 = Unbundle By Name(w646) -> ("STS"=w647:dbl)
                    n410 = Search 1D Array(1D array=w650, element="S.T.S. (V/decade):") -> (index of element=w655:i32)  [unwired: 1 in]
                    n411 = Divide(x=w655, y=3) -> (x/y=w656:dbl)
                    n412 = To Word Integer(number=w656) -> (16bit integer=w648:i16)
                    n413 = Format Value(format string="%#g", value (0)=w647) -> (output string=w659:string)  [unwired: 1 in]
                    n414 = Build Array(w649, w659) -> (w654:string[])
                    n415 = Replace Array Subset(array=w651, new element=w654, index (row)=w648) -> (w652:string[][])  [unwired: 1 in]
                  }
                }
                n416 = local write "Save Array"(w631) -> ()
              }
              frame #12 {
                w660 = "Trap Density-VT (Traps/Vcm^2):"
                n417 = local read "Save Array"() -> (w662:string[][])
                n418 = Array Size(array=w662) -> (size(s)=w667:i32[])
                n419 = Array Subset(array=w662, index (row)=0, index (col)=0, length (col)=3) -> (w663:string[][])  [unwired: 1 in]
                n420 = Index Array(array=w667, index=0) -> (element=w669:i32)
                n421 = Reshape Array(w663, w669) -> (w661:string[])
                n422 = Search 1D Array(1D array=w661, element=w660) -> (index of element=w672:i32)  [unwired: 1 in]
                n423 = Equal?(x=w672, y=-1) -> (x = y?=w671:bool)
                n424 = case shown="True" w671 {
                  tunnel: w662 -> [w682 w689]
                  tunnel: w672 -> [w678 _]
                  tunnel: [w677 w690] -> w670
                  tunnel: w661 -> [_ w688]
                  tunnel: w660 -> [_ w687]
                  frame False {
                    n425 = local read "Re-Calculated Values Cluster"() -> (w675:T8)
                    n426 = Unbundle By Name(w675) -> ("Trap Density-VT"=w674:dbl)
                    n427 = Divide(x=w678, y=3) -> (x/y=w681:dbl)
                    n428 = To Word Integer(number=w681) -> (16bit integer=w680:i16)
                    n429 = Format Value(format string="%#g", value (0)=w674) -> (output string=w679:string)  [unwired: 1 in]
                    n430 = Replace Array Subset(array=w682, new element=w679, index (row)=w680, index (col)=1) -> (w677:string[][])
                  }
                  frame True {
                    n431 = local read "Re-Calculated Values Cluster"() -> (w686:T8)
                    n432 = Unbundle By Name(w686) -> ("Trap Density-VT"=w685:dbl)
                    n433 = Search 1D Array(1D array=w688, element="STS-Sat (V/decade):") -> (index of element=w695:i32)  [unwired: 1 in]
                    n434 = Divide(x=w695, y=3) -> (x/y=w694:dbl)
                    n435 = To Word Integer(number=w694) -> (16bit integer=w696:i16)
                    n436 = Format Value(format string="%#g", value (0)=w685) -> (output string=w691:string)  [unwired: 1 in]
                    n437 = Build Array(w687, w691) -> (w698:string[])
                    n438 = Increment(x=w696) -> (x+1=w697:i16)
                    n439 = Insert Into Array(array=w689, index (row)=w697, new element=w698) -> (w690:string[][])  [unwired: 1 in]
                  }
                }
                n440 = local write "Save Array"(w670) -> ()
              }
              frame #13 {
                w700 = "Trap Density-STS (Traps/Vcm^2):"
                n441 = local read "Save Array"() -> (w702:string[][])
                n442 = Array Size(array=w702) -> (size(s)=w707:i32[])
                n443 = Array Subset(array=w702, index (row)=0, index (col)=0, length (col)=3) -> (w703:string[][])  [unwired: 1 in]
                n444 = Index Array(array=w707, index=0) -> (element=w709:i32)
                n445 = Reshape Array(w703, w709) -> (w701:string[])
                n446 = Search 1D Array(1D array=w701, element=w700) -> (index of element=w712:i32)  [unwired: 1 in]
                n447 = Equal?(x=w712, y=-1) -> (x = y?=w711:bool)
                n448 = case shown="True" w711 {
                  tunnel: w702 -> [w722 w729]
                  tunnel: w712 -> [w719 _]
                  tunnel: [w718 w730] -> w710
                  tunnel: w701 -> [_ w728]
                  tunnel: w700 -> [_ w727]
                  frame False {
                    n449 = local read "Re-Calculated Values Cluster"() -> (w715:T8)
                    n450 = Unbundle By Name(w715) -> ("Trap Density-STS"=w714:dbl)
                    n451 = Divide(x=w719, y=3) -> (x/y=w721:dbl)
                    n452 = To Word Integer(number=w721) -> (16bit integer=w720:i16)
                    n453 = Format Value(format string="%#g", value (0)=w714) -> (output string=w716:string)  [unwired: 1 in]
                    n454 = Replace Array Subset(array=w722, new element=w716, index (row)=w720, index (col)=1) -> (w718:string[][])
                  }
                  frame True {
                    n455 = local read "Re-Calculated Values Cluster"() -> (w726:T8)
                    n456 = Unbundle By Name(w726) -> ("Trap Density-STS"=w725:dbl)
                    n457 = Search 1D Array(1D array=w728, element="Trap Density-VT (Traps/Vcm^2):") -> (index of element=w735:i32)  [unwired: 1 in]
                    n458 = Divide(x=w735, y=3) -> (x/y=w736:dbl)
                    n459 = To Word Integer(number=w736) -> (16bit integer=w734:i16)
                    n460 = Format Value(format string="%#g", value (0)=w725) -> (output string=w739:string)  [unwired: 1 in]
                    n461 = Build Array(w727, w739) -> (w732:string[])
                    n462 = Increment(x=w734) -> (x+1=w733:i16)
                    n463 = Insert Into Array(array=w729, index (row)=w733, new element=w732) -> (w730:string[][])  [unwired: 1 in]
                  }
                }
                n464 = local write "Save Array"(w710) -> ()
              }
            }
            n465 = local read "New: Temp"() -> (w247:dbl)
            n466 = local read "New: Width"() -> (w248:dbl)
            n467 = local read "New: Length"() -> (w250:dbl)
            n468 = local read "Index"() -> (w249:string)
            n469 = To Single Precision Float(number=w247) -> (single precision float=w264:sgl)
            n470 = Number To Decimal String(number=w264) -> (decimal integer string=w259:string)  [unwired: 1 in]
            n471 = To Single Precision Float(number=w248) -> (single precision float=w263:sgl)
            n472 = To Single Precision Float(number=w250) -> (single precision float=w262:sgl)
            n473 = Strip Path(path=w246) -> (stripped path=w251:path)  [unwired: 1 out]
            n474 = Number To Decimal String(number=w262) -> (decimal integer string=w257:string)  [unwired: 1 in]
            n475 = Number To Decimal String(number=w263) -> (decimal integer string=w256:string)  [unwired: 1 in]
            n476 = Concatenate Strings("_", w259, "K") -> (w261:string)
            n477 = call "Build Text"("Temp"=w261, "Index"=w249, "Length"=w257, "Width"=w256) -> ("Result"=w255:string)  [unwired: 10 in, 1 out]
            n478 = Path To String(path=w251) -> (string=w253:string)
            n479 = Concatenate Strings(w253, "\\", w255) -> (w254:string)
            n480 = String To Path(string=w254) -> (path=w245:path)
          }
          frame #1 {
            n481 = flat-sequence {
              tunnel: w743 -> [w745]
              tunnel: w742 -> [w744]
              tunnel: [w744] -> w741
              tunnel: w741 -> [w751]
              tunnel: w740 -> [w750]
              frame #0 {
                n482 = Equal?(x=w745, y=w744) -> (x = y?=w746:bool)
                n483 = case shown="False" w746 {
                  tunnel: w745 -> [w749 _]
                  tunnel: w744 -> [w748 _]
                  frame False {
                    n484 = Move(source path=w749, 9:TRUE, 10:w748) -> ()  [unwired: 2 in, 3 out]
                  }
                  frame True {
                  }
                }
              }
              frame #1 {
                n485 = local write "Transfer File"(w751) -> ()
                n486 = call-poly <vilib>:"Write To Spreadsheet File.vi"("2D data"=w750, "file path (dialog if empty)"=w751) -> ()  [unwired: 6 in, 1 out]
              }
            }
          }
        }
        n487 = Cluster To Array(cluster=w239) -> (array=w238:bool[])
        n488 = Boolean Array To Number(Boolean array=w238) -> (number=w237:u32)
        n489 = Equal To 0?(x=w237) -> (x = 0?=w236:bool)
        n490 = case shown="True" w236 {
          tunnel: [MegaAwesome_States."Read Data" MegaAwesome_States."No Event"] -> w235
          frame False {
          }
          frame True {
          }
        }
      }
      frame "Save Lines" {
      }
      frame "Export" {
      }
    }
    "Current State" <- w12
    "Folder Index" <- w5
    n491 = Wait (ms)(milliseconds to wait=5) -> ()  [unwired: 1 out]
    n492 = Equal?(x=w14, y=MegaAwesome_States."Exit") -> (x = y?=w15:bool)
  }
